vi "PantherScan File Path--constant.vi"(9 "Target":string, 10 "Write":bool, 11 "Path":path) -> (2 "Continue?":bool, 3 "PantherScan file Path":path)   [LabVIEW 2019, in "Panther Dashboard.lvlib" / "Project.lvclass"]
uses:
  Project.lvclass
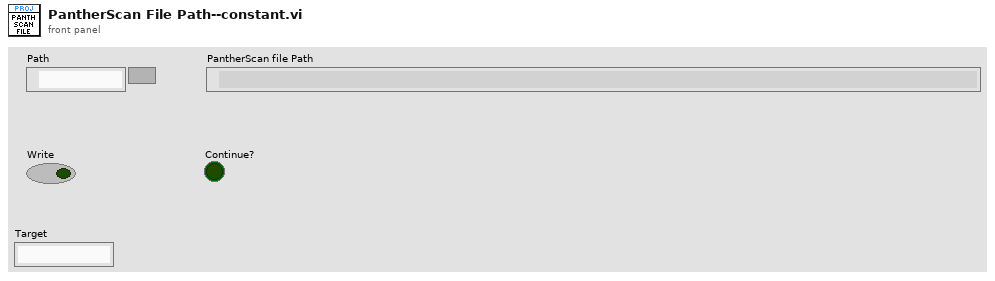
[diagram p1: front panel]
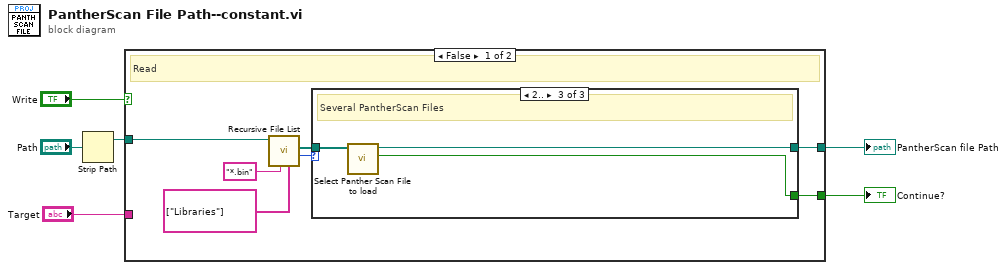
[diagram p0: block diagram]
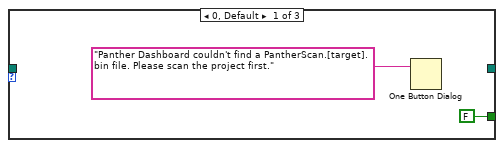
[diagram p2: hidden frame]
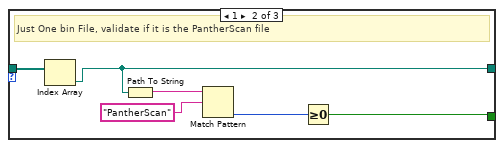
[diagram p3: hidden frame]
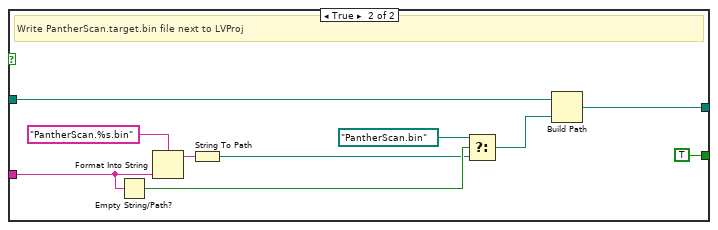
[diagram p4: hidden frame]
diagram:
  n1 = Strip Path(path="Path") -> (stripped path=w3:path)  [unwired: 1 out]
  n2 = case shown="False" "Write" {
    tunnel: [w9 w34] -> w6
    tunnel: w3 -> [w13 w31]
    tunnel: [w8 TRUE] -> w2
    tunnel: "Target" -> [_ w25]
    frame False {
      # "Read"
      n3 = call <vilib>:"Recursive File List.vi"("Folders to Exclude"=string[] ["Libraries"], "pattern"="*.bin", "Folder Path"=w13) -> ("Number of Files"=w11:i32, "All Files in Dir"=w10:path[])  [unwired: 4 in, 3 out]
      n4 = case shown="2.." w11 {
        tunnel: w10 -> [_ w21 w22]
        tunnel: [_ w20 w24] -> w9
        tunnel: [FALSE w17 w23] -> w8
        frame 0, Default {
          n5 = One Button Dialog(message="Panther Dashboard couldn't find a PantherScan.[target].bin file. Please scan the project first.") -> ()  [unwired: 1 in, 1 out]
        }
        frame 1 {
          # "Just One bin File, validate if it is the PantherScan file"
          n6 = Index Array(array=w21) -> (element=w20:path)  [unwired: 1 in]
          n7 = Path To String(path=w20) -> (string=w19:string)
          n8 = Match Pattern(string=w19, regular expression="PantherScan") -> (offset past match=w18:i32)  [unwired: 1 in, 3 out]
          n9 = Greater Or Equal To 0?(x=w18) -> (x >= 0?=w17:bool)
        }
        frame 2.. {
          # "Several PantherScan Files"
          n10 = call "Select Panther Scan File to load.vi"("PantherScan bin Files"=w22) -> ("Continue?"=w23:bool, "Panther Scan Selected"=w24:path)  [unwired: 9 in]
        }
      }
    }
    frame True {
      # "Write PantherScan.target.bin file next to LVProj"
      n11 = Empty String/Path?(string/path=w25) -> (empty?=w29:bool)
      n12 = Format Into String(format string="PantherScan.%s.bin", w25) -> (resulting string=w32:string)  [unwired: 2 in, 1 out]
      n13 = String To Path(string=w32) -> (path=w28:path)
      n14 = Select(t=path "PantherScan.bin", s=w29, f=w28) -> (s? t:f=w27:path)
      n15 = Build Path(base path=w31, name or relative path=w27) -> (appended path=w34:path)
    }
  }
  "PantherScan file Path" <- w6
  "Continue?" <- w2
